vi "Test Project Produces only one Suite from Factory method.vi"(8 "error in (no error)":errorcluster, 11 "Test Case In":refnum<class "Test FInder Test.lvclass">) -> (0 "error out":errorcluster, 3 "Test Case Out":refnum<class "Test FInder Test.lvclass">)   [LabVIEW 2020, in "Test FInder Test.lvclass"]
uses:
  Test FInder Test.lvclass
  C:/Program Files (x86)/National Instruments/LabVIEW 2020/vi.lib/Astemes/LUnit/Test Case.lvclass
  Core/Result/Type.ctl
  <vilib>/Astemes/LUnit/Test Case.lvclass/Test Case.ctl
  4ee1ff36-f2a2-4d81-80da-2416f687ba87.vi
  <vilib>/Astemes/LUnit/Palette/Pass.vi
  <vilib>/Astemes/LUnit/Palette/Fail.vi
  <vilib>/Astemes/LUnit/Compare Variants.vi
  <vilib>/Astemes/LUnit/Describe Comparison.vi
  <vilib>/Astemes/LUnit/Set Assertion Type.vi
  <vilib>/Astemes/LUnit/Add test result.vi
  <vilib>/Astemes/LUnit/Variant to string.vi
  <vilib>/Astemes/LUnit/LUnit Record Assertion Result.vi
  <vilib>/Astemes/LUnit/LUnit Aggregate Assertion Results.vi
  <vilib>/Astemes/LUnit/Method Result/LUnit Merge Status.vi
  <vilib>/Astemes/LUnit/LUnit Concatenate result strings.vi
  <vilib>/Utility/Data Type/Get Type Information.vi
  <vilib>/Utility/LVClass/Get LV Class Name.vi
  Core/LUnit Test Suite/LUnit Test Suite.lvclass
  Test FInder Test.lvclass/Test FInder Test.ctl
  Core/Result/Result.lvlib
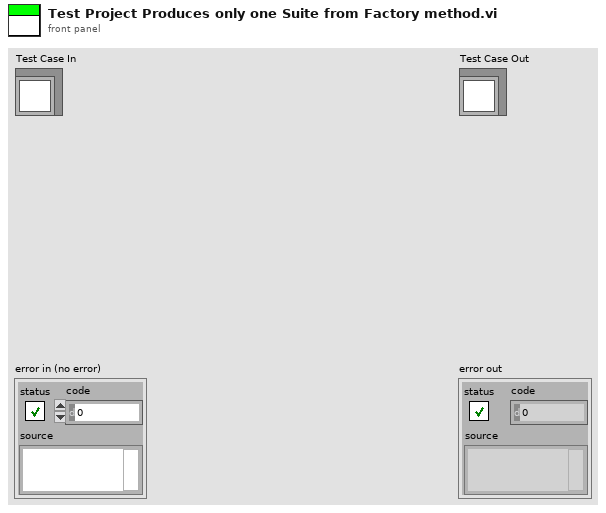
[diagram p1: front panel]
types:
  T1 = typedef "Result.lvlib/Result.ctl" = cluster{"Name":string, "Message":string, "Description":string, "Status":T2, "Result Type":T3, "Execution Time":dbl}
  T2 = typedef "Result.lvlib/Status.ctl" = enum16{"", "Passed", "Failed", "Error", "Skipped", "Setup Error", "Broken", "Teardown Error"}
  T3 = typedef "Result.lvlib/Type.ctl" = enum16{"Method", "Case", "Suite", "Pass", "Fail", "Skip", "Pass if", "Fail if", "Pass if Error", "Fail if Error", "Pass if Equal", "Fail if Equal"}
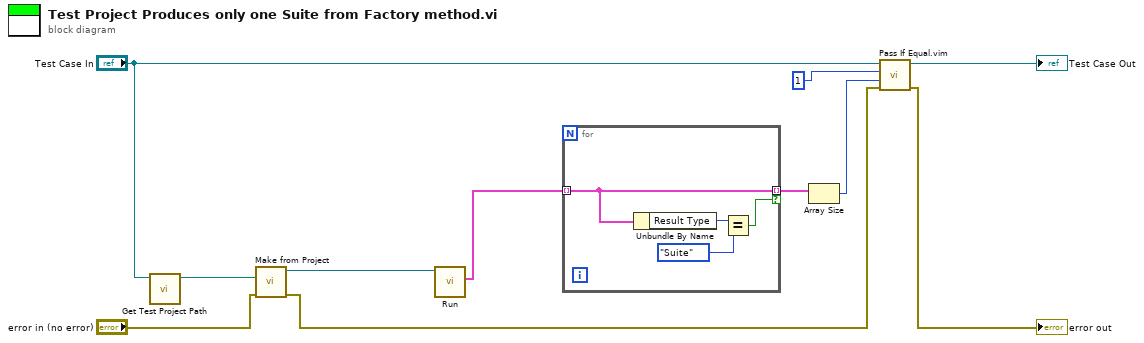
[diagram p0: block diagram]
diagram:
  n1 = call "Get Test Project Path.vi"("LUnit Test Suite Tests in"="Test Case In") -> ("appended path"=w8:path)  [unwired: 10 in]
  n2 = call "Make from Project.vi"("error in (no error)"="error in (no error)", "Project Path"=w8) -> ("error out"=w9:errorcluster, "LUnit Test Suite Out"=w7:refnum<class "LUnit Test Suite.lvclass">)  [unwired: 8 in]
  n3 = call-dynamic "Run.vi"("LUnit Test Suite In"=w7) -> ("Results"=w3:T1[])  [unwired: 9 in, 1 out]
  n4 = for {
    tunnel: w3 -> [w13] mode=indexing
    tunnel: [w13] -> w4 mode=indexing if=w12
    n5 = Unbundle By Name(w13) -> ("Result Type"=w15:T3)
    n6 = Equal?(x=w15, y=Type."Suite") -> (x = y?=w12:bool)
  }
  n7 = Array Size(array=w4) -> (size(s)=w2:i32)
  n8 = call "Pass If Equal.vim"("error in (no error)"=w9, "Actual"=w2, "Expected"=1 ("size(s)"), "LUnit Test Case In"="Test Case In") -> ("error out"=→"error out":errorcluster, "LUnit Test Case Out"=→"Test Case Out":refnum<class "Test FInder Test.lvclass">)  [unwired: 6 in]
